vi "read_OSC.vi"(5 "Channel (0: Channel 1)":u16(ring)=1 items=["Channel 1", "Channel 2", "Channel 3", "Channel 4", "Math 1", "Math 2", "Math 3", "Math 4", "Reference 1", "Reference 2", "Reference 3", "Reference 4"], 11 "error in (no error)":errorcluster) -> (1 "raw Waveform Data":waveform(dbl)(graph)={"t0"=timestamp(1.815305999999491e-07 s since 1904-01-01), "dt"=5e-07, "Y"=array[10000 elements]}, 2 "t0":timestamp, 3 "dt":dbl, 4 "VISA resource name out":refnum<visa-resource-name>, 12 "ave. background TD signal":dbl[](array[numeric]), 13 "ave. molecularTD signal":dbl[](array[numeric]), 14 "cor. ave. TD signal":dbl[](array[numeric]), 15 "error out":errorcluster)   [LabVIEW 2011]
doc: "Demonstrates how to set up an oscilloscope automatically. You can configure this VI to acquire a waveform from a single channel by following the following steps:\n\n1. Specify a valid VISA resource to use. \n2. Specify a channel. \n3. Specify a time-out value for reading a waveform.\n4. Run this VI. The <B>Waveform Graph</B> displays the waveform you acquire."
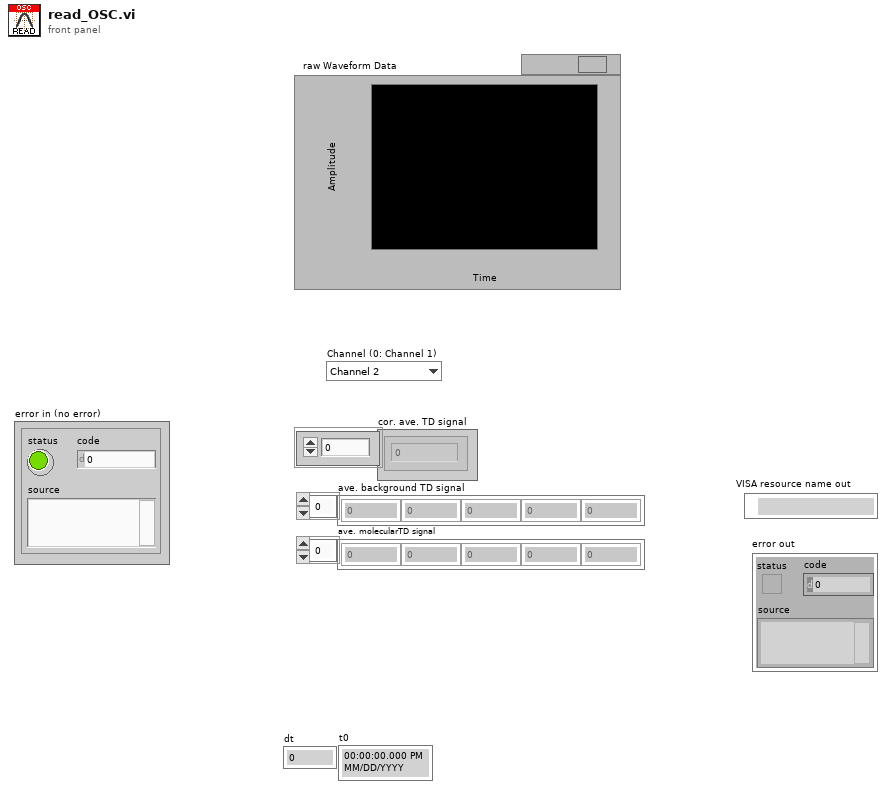
[diagram p1: front panel]
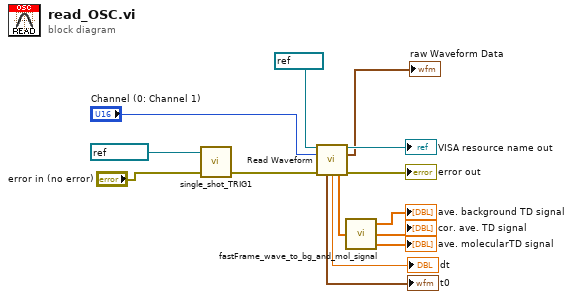
[diagram p0: block diagram]
diagram:
  n1 = call "single_shot_TRIG1.vi"("error in (no error)"="error in (no error)", "VISA resource name"=refnum<visa-resource-name> "TRIG1") -> ("error out"=w13:errorcluster)  [unwired: 2 in, 1 out]
  n2 = call "Read Waveform.vi"("VISA resource name"=refnum<visa-resource-name> "OSC", "Channel (0: Channel 1)"="Channel (0: Channel 1)", "error in (no error)"=w13) -> ("VISA resource name out"=→"VISA resource name out":refnum<visa-resource-name>, "Waveform Data"=→"raw Waveform Data":waveform(dbl), "t0"=→"t0":timestamp, "dt"=→"dt":dbl, "raw array data"=w11:dbl[], "error out"=→"error out":errorcluster)  [unwired: 7 in]
  n3 = call "fastFrame_wave_to_bg_and_mol_signal.vi"("all fast frames"=w11) -> ("ave. molecularTD signal"=→"ave. molecularTD signal":dbl[], "cor. ave. TD signal"=→"cor. ave. TD signal":dbl[], "ave. background TD signal"=→"ave. background TD signal":dbl[])  [unwired: 2 in]
